vi "Tree Filter.vi"(7 "Boolean Connectors":string[](array[string]), 8 "error in":errorcluster, 9 "Comparators":T2(array[cluster]), 10 "Headers":string[](array[string]), 11 "Frame groups":T1(array[cluster])) -> (0 "error out":errorcluster, 3 "Filtered tree":string[][](array[string]))   [LabVIEW 2025, in "CAN-LIN Raw Bus Capture UI.lvlib"]
uses:
  CAN-LIN Raw Bus Capture UI.lvlib
  Table_Filtering/Table_Filtering.lvlib
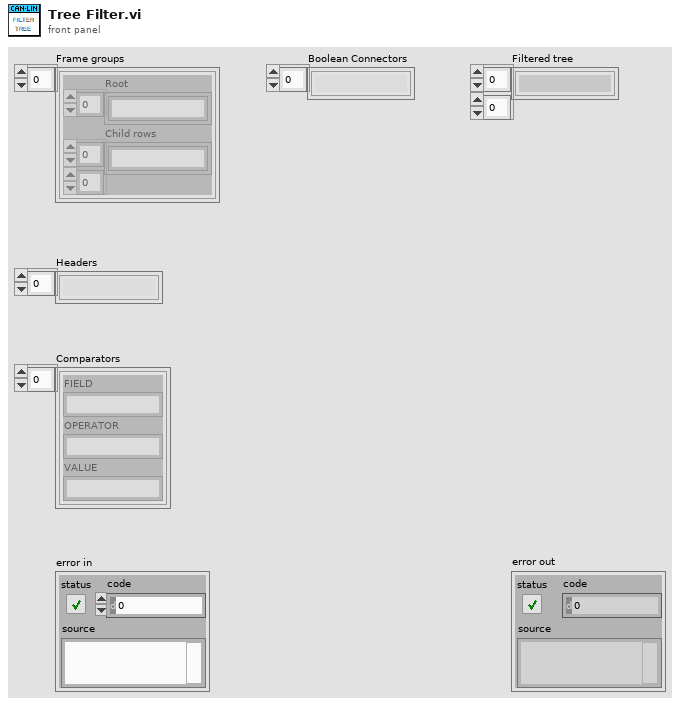
[diagram p1: front panel]
types:
  T1 = cluster{"Root":string[], "Child rows":string[][]}[]
  T2 = cluster{"FIELD":string, "OPERATOR":string, "VALUE":string}[]
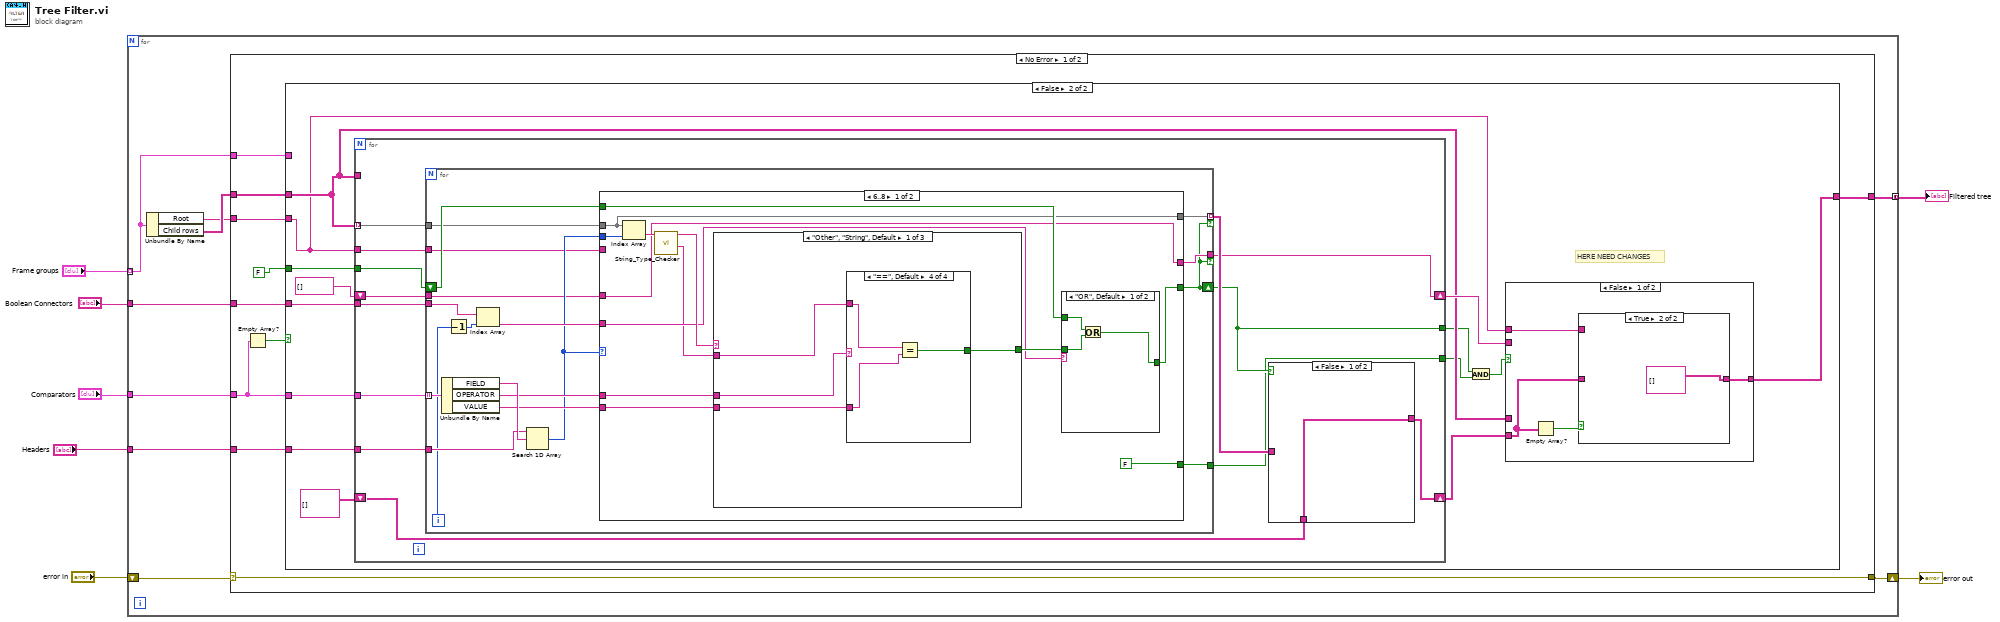
[diagram p0: block diagram]
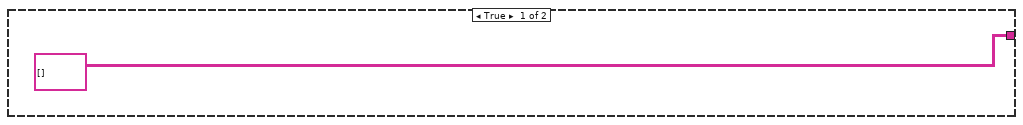
[diagram p2: hidden frame]
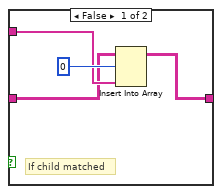
[diagram p3: hidden frame]
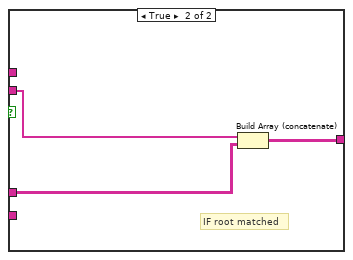
[diagram p4: hidden frame]
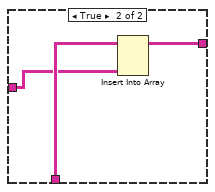
[diagram p5: hidden frame]
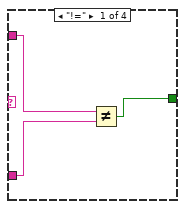
[diagram p6: hidden frame]
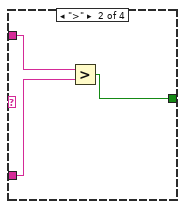
[diagram p7: hidden frame]
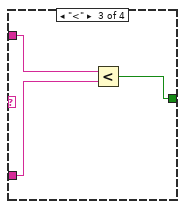
[diagram p8: hidden frame]
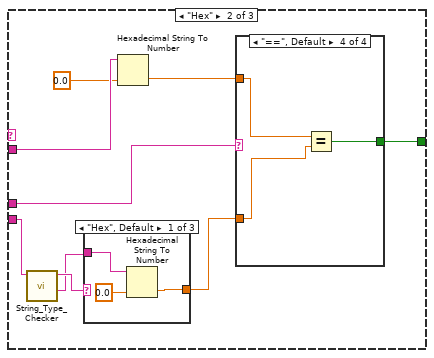
[diagram p9: hidden frame]
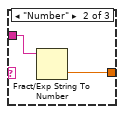
[diagram p10: hidden frame]
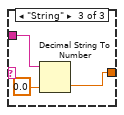
[diagram p11: hidden frame]
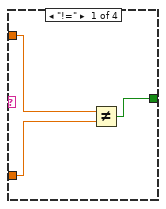
[diagram p12: hidden frame]
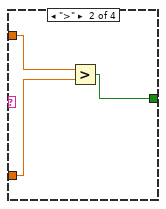
[diagram p13: hidden frame]
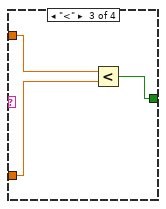
[diagram p14: hidden frame]
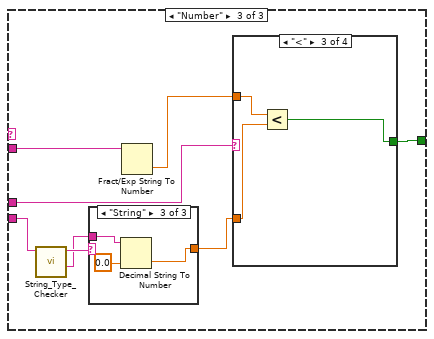
[diagram p15: hidden frame]
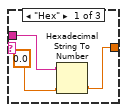
[diagram p16: hidden frame]
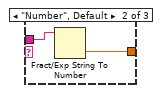
[diagram p17: hidden frame]
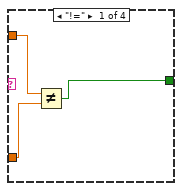
[diagram p18: hidden frame]
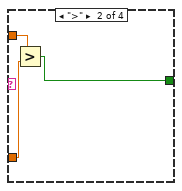
[diagram p19: hidden frame]
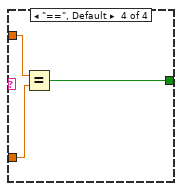
[diagram p20: hidden frame]
diagram:
  n1 = for {
    tunnel: "Frame groups" -> [w10] mode=indexing
    tunnel: "Comparators" -> [w16]
    tunnel: "Boolean Connectors" -> [w15]
    tunnel: "Headers" -> [w13]
    tunnel: [w11] -> w7 mode=concatenating
    shift-right: [w9] -> w2
    shift-left: "error in" -> [w8]
    n2 = Unbundle By Name(w10) -> ("Root"=w12:string[], "Child rows"=w14:string[][])
    n3 = case shown="No Error" w8 {
      selector: w8 -> [w22 w273]
      tunnel: w13 -> [w26 _]
      tunnel: w15 -> [w25 _]
      tunnel: w16 -> [w19 _]
      tunnel: w14 -> [w24 _]
      tunnel: [w23 _] -> w11
      tunnel: [w22 w273] -> w9
      tunnel: w12 -> [w18 _]
      tunnel: w10 -> [w17 _]
      frame No Error {
        n4 = Empty Array?(array=w19) -> (empty?=w20:bool)
        n5 = case shown="False" w20 {
          tunnel: w26 -> [_ w41]
          tunnel: FALSE -> [_ w40]
          tunnel: w25 -> [_ w39]
          tunnel: w19 -> [_ w38]
          tunnel: w24 -> [_ w34]
          tunnel: [string[][] [] ("Child rows") w35] -> w23
          tunnel: w18 -> [_ w28]
          tunnel: w17 -> [_ _]
          frame True {
          }
          frame False {
            # "HERE NEED CHANGES"
            n6 = for {
              tunnel: w41 -> [w66]
              tunnel: w38 -> [w65]
              tunnel: w34 -> [w62] mode=indexing
              tunnel: w40 -> [w64]
              tunnel: w39 -> [w63]
              tunnel: w28 -> [w58]
              tunnel: w34 -> [_]
              shift-right: [w61] -> w33
              shift-left: string[][] [] -> [w59]
              tunnel: [w57] -> w31
              tunnel: [w56] -> w30
              shift-right: [w54] -> w36
              shift-left: string[] [] ("Root") -> [w55]
              n7 = for {
                tunnel: w66 -> [w86]
                tunnel: w65 -> [w88] mode=indexing
                tunnel: w62 -> [w76]
                shift-right: [w71] -> w57
                shift-left: w64 -> [w82]
                tunnel: w63 -> [w85]
                tunnel: w58 -> [w77]
                tunnel: [w75] -> w56
                tunnel: [w74] -> w60 mode=indexing if=w71
                tunnel: w55 -> [w73]
                tunnel: [w72] -> w54 if=w71
                i -> [w83]
                n8 = Unbundle By Name(w88) -> ("FIELD"=w87:string, "OPERATOR"=w80:string, "VALUE"=w81:string)
                n9 = Decrement(x=w83) -> (x-1=w84:i32)
                n10 = Index Array(array=w85, index=w84) -> (element=w79:string)
                n11 = Search 1D Array(1D array=w86, element=w87) -> (index of element=w78:i32)  [unwired: 1 in]
                n12 = case shown="6..8" w78 {
                  tunnel: w76 -> [w90 _]
                  tunnel: w78 -> [w101 w193]
                  tunnel: w82 -> [w100 w192]
                  tunnel: [w92 w191] -> w71
                  tunnel: w81 -> [w97 w188]
                  tunnel: w80 -> [w96 w187]
                  tunnel: w79 -> [w94 w185]
                  tunnel: w77 -> [_ w181]
                  tunnel: [FALSE ("Root row?") w183] -> w75
                  tunnel: [w90 string[] [] ("Child rows")] -> w74
                  tunnel: w73 -> [w89 _]
                  tunnel: [w89 w181] -> w72
                  frame 6..8 {
                    n13 = Index Array(array=w90, index=w101) -> (element=w98:string)
                    n14 = call "String_Type_Checker.vi"("String"=w98) -> ("Number"=w93:string, "Type"=w99:string)  [unwired: 9 in]
                    n15 = case shown="\"Other\", \"String\", Default" w99 {
                      tunnel: w93 -> [w105 w126 w154]
                      tunnel: w97 -> [w102 w121 w150]
                      tunnel: w96 -> [w104 w124 w153]
                      tunnel: [w103 w123 w152] -> w95
                      frame "Other", "String", Default {
                        n16 = case shown="\"==\", Default" w104 {
                          tunnel: w105 -> [w107 w111 w114 w115]
                          tunnel: w102 -> [w106 w110 w113 w117]
                          tunnel: [w108 w109 w112 w116] -> w103
                          frame "!=" {
                            n17 = Not Equal?(x=w107, y=w106) -> (x != y?=w108:bool)
                          }
                          frame ">" {
                            n18 = Greater?(x=w111, y=w110) -> (0:w109:bool)
                          }
                          frame "<" {
                            n19 = Less?(x=w114, y=w113) -> (x < y?=w112:bool)
                          }
                          frame "==", Default {
                            n20 = Equal?(x=w115, y=w117) -> (x = y?=w116:bool)
                          }
                        }
                      }
                      frame "Hex" {
                        n21 = call "String_Type_Checker.vi"("String"=w121) -> ("Number"=w118:string, "Type"=w119:string)  [unwired: 9 in]
                        n22 = case shown="\"Hex\", Default" w119 {
                          tunnel: [w127 w131 w134] -> w122
                          tunnel: w118 -> [w129 w130 w132]
                          frame "Hex", Default {
                            n23 = Hexadecimal String To Number(string=w129, default (0uL)=0.0) -> (number=w127:dbl)  [unwired: 1 in, 1 out]
                          }
                          frame "Number" {
                            n24 = Fract/Exp String To Number(string=w130) -> (number=w131:dbl)  [unwired: 3 in, 1 out]
                          }
                          frame "String" {
                            n25 = Decimal String To Number(string=w132, default (0L)=0.0) -> (number=w134:dbl)  [unwired: 1 in, 1 out]
                          }
                        }
                        n26 = Hexadecimal String To Number(string=w126, default (0uL)=0.0) -> (number=w125:dbl)  [unwired: 1 in, 1 out]
                        n27 = case shown="\"==\", Default" w124 {
                          tunnel: w125 -> [w136 w140 w143 w144]
                          tunnel: w122 -> [w135 w139 w142 w146]
                          tunnel: [w137 w138 w141 w145] -> w123
                          frame "!=" {
                            n28 = Not Equal?(x=w136, y=w135) -> (x != y?=w137:bool)
                          }
                          frame ">" {
                            n29 = Greater?(x=w140, y=w139) -> (0:w138:bool)
                          }
                          frame "<" {
                            n30 = Less?(x=w143, y=w142) -> (x < y?=w141:bool)
                          }
                          frame "==", Default {
                            n31 = Equal?(x=w144, y=w146) -> (x = y?=w145:bool)
                          }
                        }
                      }
                      frame "Number" {
                        n32 = call "String_Type_Checker.vi"("String"=w150) -> ("Number"=w148:string, "Type"=w149:string)  [unwired: 9 in]
                        n33 = case shown="\"String\"" w149 {
                          tunnel: [w155 w159 w162] -> w147
                          tunnel: w148 -> [w157 w158 w160]
                          frame "Hex" {
                            n34 = Hexadecimal String To Number(string=w157, default (0uL)=0.0) -> (number=w155:dbl)  [unwired: 1 in, 1 out]
                          }
                          frame "Number", Default {
                            n35 = Fract/Exp String To Number(string=w158) -> (number=w159:dbl)  [unwired: 3 in, 1 out]
                          }
                          frame "String" {
                            n36 = Decimal String To Number(string=w160, default (0L)=0.0) -> (number=w162:dbl)  [unwired: 1 in, 1 out]
                          }
                        }
                        n37 = Fract/Exp String To Number(string=w154) -> (number=w151:dbl)  [unwired: 3 in, 1 out]
                        n38 = case shown="\"<\"" w153 {
                          tunnel: w147 -> [w164 w168 w171 w174]
                          tunnel: [w165 w167 w170 w173] -> w152
                          tunnel: w151 -> [w163 w166 w169 w172]
                          frame "!=" {
                            n39 = Not Equal?(x=w163, y=w164) -> (x != y?=w165:bool)
                          }
                          frame ">" {
                            n40 = Greater?(x=w166, y=w168) -> (0:w167:bool)
                          }
                          frame "<" {
                            n41 = Less?(x=w169, y=w171) -> (x < y?=w170:bool)
                          }
                          frame "==", Default {
                            n42 = Equal?(x=w172, y=w174) -> (x = y?=w173:bool)
                          }
                        }
                      }
                    }
                    n43 = case shown="\"OR\", Default" w94 {
                      tunnel: w100 -> [w176 w180]
                      tunnel: [w177 w179] -> w92
                      tunnel: w95 -> [w175 w178]
                      frame "OR", Default {
                        n44 = Or(x=w176, y=w175) -> (x .or. y?=w177:bool)
                      }
                      frame "AND" {
                        n45 = And(x=w180, y=w178) -> (x .and. y?=w179:bool)
                      }
                    }
                  }
                  frame 0..5, Default {
                    w183 = TRUE  # Root row?
                    n46 = Index Array(array=w181, index=w193) -> (element=w189:string)
                    n47 = call "String_Type_Checker.vi"("String"=w189) -> ("Number"=w184:string, "Type"=w190:string)  [unwired: 9 in]
                    n48 = case shown="\"Number\"" w190 {
                      tunnel: w184 -> [w197 w218 w246]
                      tunnel: w188 -> [w194 w213 w242]
                      tunnel: w187 -> [w196 w216 w245]
                      tunnel: [w195 w215 w244] -> w186
                      frame "Other", "String", Default {
                        n49 = case shown="\">\"" w196 {
                          tunnel: w197 -> [w199 w203 w206 w207]
                          tunnel: w194 -> [w198 w202 w205 w209]
                          tunnel: [w200 w201 w204 w208] -> w195
                          frame "!=" {
                            n50 = Not Equal?(x=w199, y=w198) -> (x != y?=w200:bool)
                          }
                          frame ">" {
                            n51 = Greater?(x=w203, y=w202) -> (0:w201:bool)
                          }
                          frame "<" {
                            n52 = Less?(x=w206, y=w205) -> (x < y?=w204:bool)
                          }
                          frame "==", Default {
                            n53 = Equal?(x=w207, y=w209) -> (x = y?=w208:bool)
                          }
                        }
                      }
                      frame "Hex" {
                        n54 = call "String_Type_Checker.vi"("String"=w213) -> ("Number"=w210:string, "Type"=w211:string)  [unwired: 9 in]
                        n55 = case shown="\"Hex\", Default" w211 {
                          tunnel: [w219 w223 w226] -> w214
                          tunnel: w210 -> [w221 w222 w224]
                          frame "Hex", Default {
                            n56 = Hexadecimal String To Number(string=w221, default (0uL)=0.0) -> (number=w219:dbl)  [unwired: 1 in, 1 out]
                          }
                          frame "Number" {
                            n57 = Fract/Exp String To Number(string=w222) -> (number=w223:dbl)  [unwired: 3 in, 1 out]
                          }
                          frame "String" {
                            n58 = Decimal String To Number(string=w224, default (0L)=0.0) -> (number=w226:dbl)  [unwired: 1 in, 1 out]
                          }
                        }
                        n59 = Hexadecimal String To Number(string=w218, default (0uL)=0.0) -> (number=w217:dbl)  [unwired: 1 in, 1 out]
                        n60 = case shown="\"==\", Default" w216 {
                          tunnel: w217 -> [w228 w232 w235 w236]
                          tunnel: w214 -> [w227 w231 w234 w238]
                          tunnel: [w229 w230 w233 w237] -> w215
                          frame "!=" {
                            n61 = Not Equal?(x=w228, y=w227) -> (x != y?=w229:bool)
                          }
                          frame ">" {
                            n62 = Greater?(x=w232, y=w231) -> (0:w230:bool)
                          }
                          frame "<" {
                            n63 = Less?(x=w235, y=w234) -> (x < y?=w233:bool)
                          }
                          frame "==", Default {
                            n64 = Equal?(x=w236, y=w238) -> (x = y?=w237:bool)
                          }
                        }
                      }
                      frame "Number" {
                        n65 = call "String_Type_Checker.vi"("String"=w242) -> ("Number"=w240:string, "Type"=w241:string)  [unwired: 9 in]
                        n66 = case shown="\"Number\", Default" w241 {
                          tunnel: [w247 w251 w254] -> w239
                          tunnel: w240 -> [w249 w250 w252]
                          frame "Hex" {
                            n67 = Hexadecimal String To Number(string=w249, default (0uL)=0.0) -> (number=w247:dbl)  [unwired: 1 in, 1 out]
                          }
                          frame "Number", Default {
                            n68 = Fract/Exp String To Number(string=w250) -> (number=w251:dbl)  [unwired: 3 in, 1 out]
                          }
                          frame "String" {
                            n69 = Decimal String To Number(string=w252, default (0L)=0.0) -> (number=w254:dbl)  [unwired: 1 in, 1 out]
                          }
                        }
                        n70 = Fract/Exp String To Number(string=w246) -> (number=w243:dbl)  [unwired: 3 in, 1 out]
                        n71 = case shown="\"==\", Default" w245 {
                          tunnel: w239 -> [w256 w260 w263 w266]
                          tunnel: [w257 w259 w262 w265] -> w244
                          tunnel: w243 -> [w255 w258 w261 w264]
                          frame "!=" {
                            n72 = Not Equal?(x=w255, y=w256) -> (x != y?=w257:bool)
                          }
                          frame ">" {
                            n73 = Greater?(x=w258, y=w260) -> (0:w259:bool)
                          }
                          frame "<" {
                            n74 = Less?(x=w261, y=w263) -> (x < y?=w262:bool)
                          }
                          frame "==", Default {
                            n75 = Equal?(x=w264, y=w266) -> (x = y?=w265:bool)
                          }
                        }
                      }
                    }
                    n76 = case shown="\"OR\", Default" w185 {
                      tunnel: w192 -> [w268 w272]
                      tunnel: [w269 w271] -> w191
                      tunnel: w186 -> [w267 w270]
                      frame "OR", Default {
                        n77 = Or(x=w268, y=w267) -> (x .or. y?=w269:bool)
                      }
                      frame "AND" {
                        n78 = And(x=w272, y=w270) -> (x .and. y?=w271:bool)
                      }
                    }
                  }
                }
              }
              n79 = case shown="False" w57 {
                tunnel: [w67 w68] -> w61
                tunnel: w60 -> [_ w69]
                tunnel: w59 -> [w67 w70]
                frame False {
                }
                frame True {
                  n80 = Insert Into Array(array=w70, new element=w69) -> (w68:string[][])  [unwired: 2 in]
                }
              }
            }
            n81 = And(x=w31, y=w30) -> (x .and. y?=w32:bool)
            n82 = case shown="False" w32 {
              tunnel: w36 -> [_ w53]
              tunnel: [w45 w51] -> w35
              tunnel: w34 -> [_ w52]
              tunnel: w33 -> [w43 _]
              tunnel: w28 -> [w44 _]
              frame False {
                n83 = Empty Array?(array=w43) -> (empty?=w42:bool)
                n84 = case shown="True" w42 {
                  tunnel: [w49 string[][] []] -> w45
                  tunnel: w44 -> [w47 _]
                  tunnel: w43 -> [w46 _]
                  frame False {
                    # "If child matched"
                    n85 = Insert Into Array(array=w46, index (row)=0, new element=w47) -> (w49:string[][])  [unwired: 1 in]
                  }
                  frame True {
                  }
                }
              }
              frame True {
                # "IF root matched"
                n86 = Build Array (concatenate)(w53, w52) -> (w51:string[][])
              }
            }
          }
        }
      }
      frame Error {
      }
    }
  }
  "Filtered tree" <- w7
  "error out" <- w2
